vi "Polymorphic - Read LineFeed Terminated String.vi"   [LabVIEW 2021]
doc: "Read data from the connection to the DAQiFi device, 1 byte at a time, until the newline character is encountered.\n\nThe newline character marks the end of the transmission."
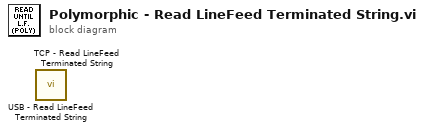
[diagram p0: block diagram]
diagram:
  n1 = call "USB - Read LineFeed Terminated String.vi"() -> ()  [unwired: 9 in, 3 out]
  n2 = call "TCP - Read LineFeed Terminated String.vi"() -> ()  [unwired: 9 in, 3 out]
